vi "Data_Xml_Spectrum_Names.vi"(7 "Acquisition Number":i16, 8 "error in (no error)":errorcluster, 11 "QMH ICR Cluster":T1) -> (0 "error out":errorcluster caption="sortie d'erreur", 3 "QMH ICR Cluster":T1)   [LabVIEW 2024]
doc: "This VI returns the next spectrum prefix available, with the naming convention yyyy_mm_dd_xxx.\nxxx is the spectrum number."
uses:
  controls/QMH_ICR_Cluster.ctl
  controls/HARDWARE_Resources.ctl
  controls/PROCESSING_Inputs.ctl
  controls/LOOPS_Inputs.ctl
  controls/OPO_Inputs.ctl
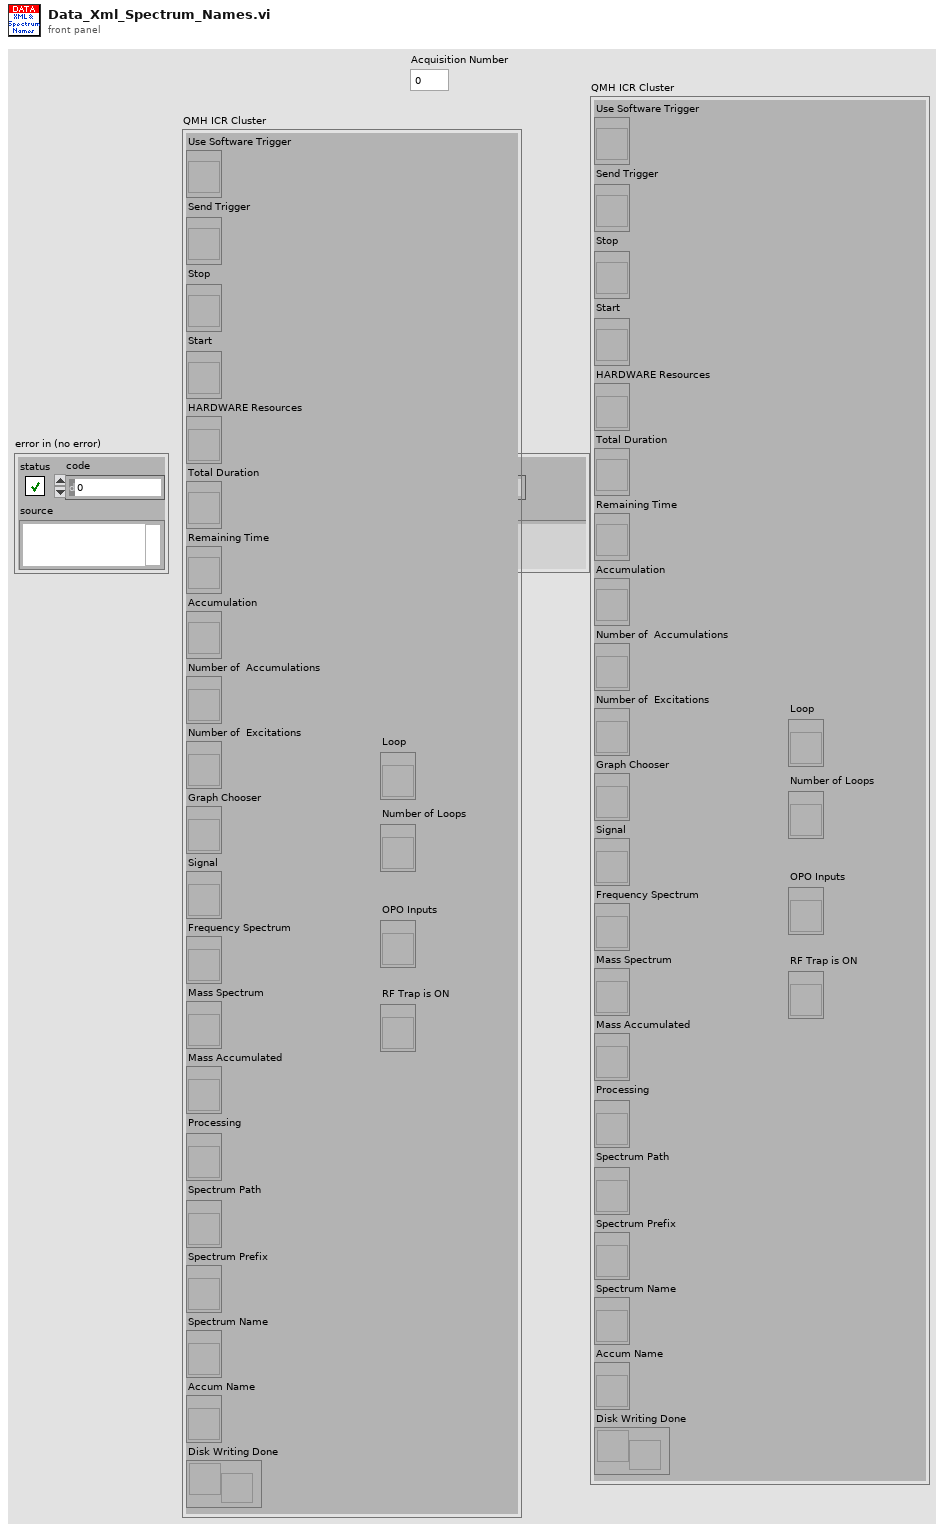
[diagram p1: front panel]
types:
  T1 = typedef "QMH_ICR_Cluster.ctl" = cluster{"Use Software Trigger":refnum<vi>, "Send Trigger":refnum<vi>, "Stop":refnum<vi>, "Start":refnum<vi>, "HARDWARE Resources":refnum<vi>, "Total Duration":refnum<vi>, "Remaining Time":refnum<vi>, "Accumulation":refnum<vi>, "Number of  Accumulations":refnum<vi>, "Number of  Excitations":refnum<vi>, "Graph Chooser":refnum<vi>, "Signal":refnum<vi>, "Frequency Spectrum":refnum<vi>, "Mass Spectrum":refnum<vi>, "Mass Accumulated":refnum<vi>, "Processing":refnum<vi>, "Spectrum Path":refnum<vi>, "Spectrum Prefix":refnum<vi>, "Spectrum Name":refnum<vi>, "Accum Name":refnum<vi>, "Disk Writing Done":refnum<notifier>, "Loop":refnum<vi>, "Number of Loops":refnum<vi>, "OPO Inputs":refnum<vi>, "RF Trap is ON":refnum<vi>}
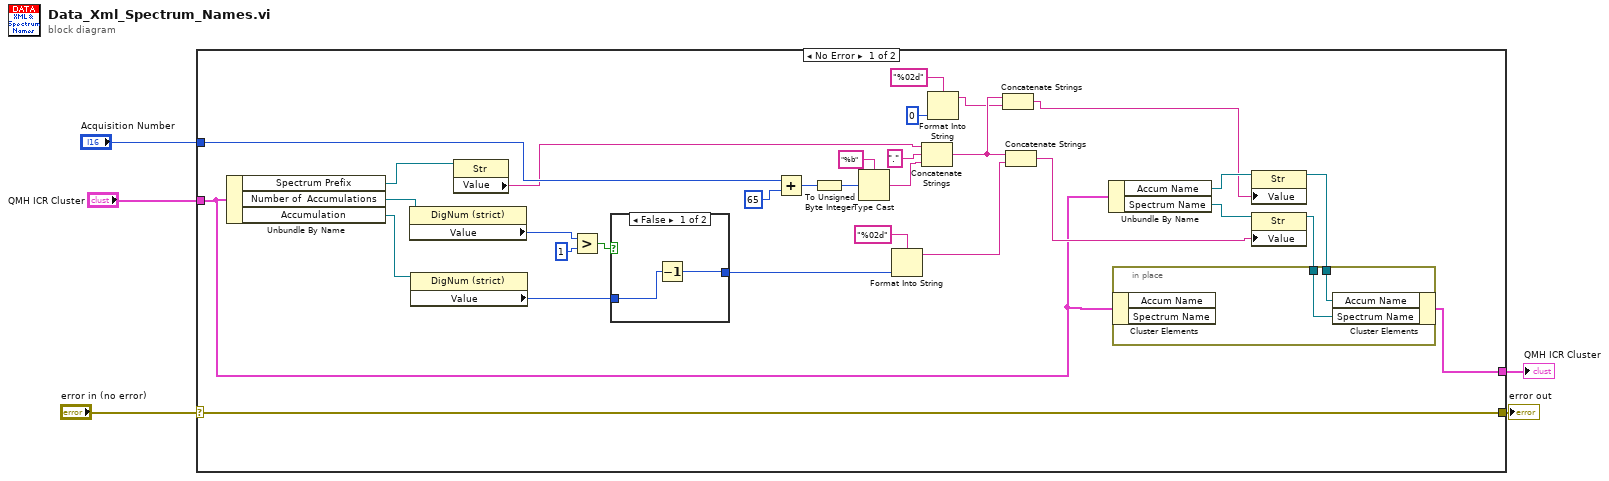
[diagram p0: block diagram]
diagram:
  n1 = case shown="No Error" "error in (no error)" {
    selector: "error in (no error)" -> [w12 w43]
    tunnel: "Acquisition Number" -> [w36 _]
    tunnel: "QMH ICR Cluster" -> [w9 w42]
    tunnel: [w12 w43] -> w2
    tunnel: [w6 w42] -> w1
    frame No Error {
      n2 = Unbundle By Name(w9) -> ("Spectrum Prefix"=w34:refnum<vi>, "Number of  Accumulations"=w35:refnum<vi>, "Accumulation"=w32:refnum<vi>)
      n3 = property class="DigNum (strict)"(reference=w35) -> ("Value"=w10:i16)  [unwired: 1 in, 2 out]
      n4 = property class="DigNum (strict)"(reference=w32) -> ("Value"=w11:i16)  [unwired: 1 in, 2 out]
      n5 = property class="Str"(reference=w34) -> ("Value"=w33:string)  [unwired: 1 in, 2 out]
      n6 = Greater?(x=w10, y=i16 1) -> (0:w24:bool)
      n7 = case shown="False" w24 {
        tunnel: [w40 w41] -> w23
        tunnel: w11 -> [w39 w41]
        frame False {
          n8 = Decrement(x=w39) -> (x-1=w40:i16)
        }
        frame True {
        }
      }
      n9 = Add(x=w36, y=i16 65) -> (x+y=w29:i16)
      n10 = To Unsigned Byte Integer(number=w29) -> (unsigned 8bit integer=w30:u8)
      n11 = Type Cast(type="%b", x=w30) -> (*(type *) &x=w27:string)
      n12 = Format Into String(format string="%02d" ("chaîne de format"), w23) -> (resulting string=w21:string)  [unwired: 2 in, 1 out]
      n13 = Concatenate Strings(w33, "." ("chaîne"), w27) -> (w18:string)
      n14 = Format Into String(format string="%02d" ("chaîne de format"), i16 0 ("entrée 1")) -> (resulting string=w17:string)  [unwired: 2 in, 1 out]
      n15 = Concatenate Strings(w18, w17) -> (w15:string)
      n16 = Concatenate Strings(w18, w21) -> (w13:string)
      n17 = Unbundle By Name(w9) -> ("Accum Name"=w16:refnum<vi>, "Spectrum Name"=w14:refnum<vi>)
      n18 = property class="Str"(reference=w16, "Value"=w15) -> (reference out=w7:refnum<vi>)  [unwired: 1 in, 1 out]
      n19 = property class="Str"(reference=w14, "Value"=w13) -> (reference out=w8:refnum<vi>)  [unwired: 1 in, 1 out]
      n20 = in-place {
        in-place-border: w8 -> [w38]
        in-place-border: w7 -> [w37]
        n21 = in-place-cluster #1(w9) -> ()  [unwired: 2 out]
        n22 = in-place-cluster #1("Accum Name"=w37, "Spectrum Name"=w38) -> (w6:T1)
      }
    }
    frame Error {
    }
  }
  "error out" <- w2
  "QMH ICR Cluster" <- w1
